vi "调用方.vi"   [LabVIEW 2018]
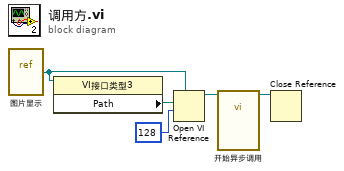
[diagram p0: block diagram]
diagram:
  n1 = vi-ref "图片显示.vi"() -> (w5:refnum<vi>)
  n2 = property class="VI接口类型3"(reference=w5) -> ("Path"=w4:path)  [unwired: 1 in, 2 out]
  n3 = Open VI Reference(type specifier VI Refnum (for type only)=w5, vi path=w4, options=128 ("选项")) -> (vi reference=w2:refnum<vi>)  [unwired: 3 in, 1 out]
  n4 = call-by-ref "开始异步调用"(reference=w2) -> (reference out=w1:refnum<vi>)  [unwired: 3 in, 1 out]
  n5 = Close Reference(reference=w1) -> ()  [unwired: 1 in, 1 out]
